vi "Assert QueryNames.vi"() -> ()   [LabVIEW 2015, in "ExcuseNotesHandler.lvclass"]
uses:
  ExcuseNotesHandler.lvclass
  API/_Database/Database.lvclass
  ExcuseNotesHandler.lvclass/ExcuseNotesHandler.ctl
panel:
  out "Names(\"\")":string[](array[string])
  in  "path":path=path "E:/哈工大竞技机器人队/机器人队管理系统/Database/CRTDatabase.accdb"
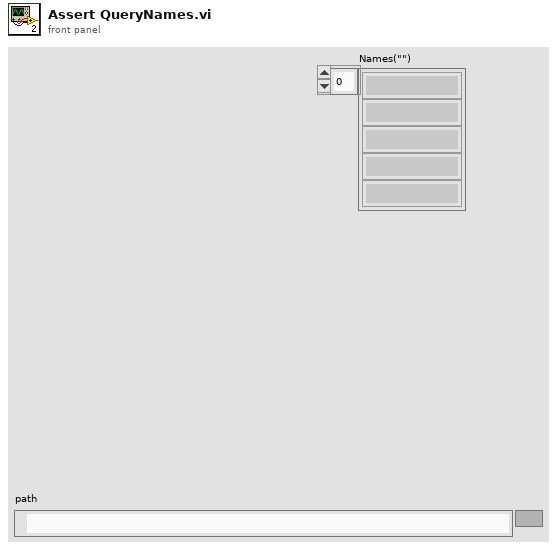
[diagram p1: front panel]
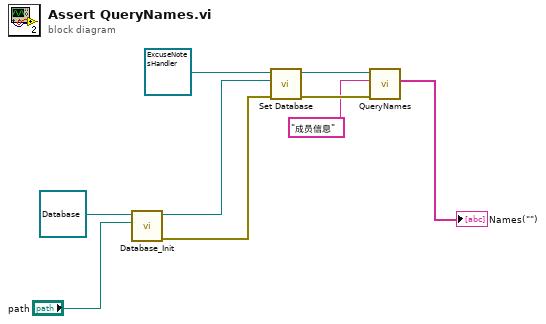
[diagram p0: block diagram]
diagram:
  n1 = call "Database_Init.vi"("path"="path", "object in"=refnum<class "Database.lvclass"> refnum ("Database")) -> ("error out"=w3:errorcluster, "object out"=w4:refnum<class "Database.lvclass">)  [unwired: 8 in]
  n2 = call "Set Database.vi"("error in (no error)"=w3, "Database"=w4, "ExcuseNotes in"=refnum<class "ExcuseNotesHandler.lvclass"> refnum ("Admin_Actor.lvlib:ExcuseNotes.lvclass")) -> ("error out"=w7:errorcluster, "ExcuseNotes out"=w8:refnum<class "ExcuseNotesHandler.lvclass">)  [unwired: 7 in]
  n3 = call "QueryNames.vi"("error in (no error)"=w7, "TableName(\"\")"="成员信息" ("TableName(\"\")"), "ExcuseNotes in"=w8) -> ("Names(\"\")"=→"Names(\"\")":string[])  [unwired: 6 in, 2 out]
